vi "S_ReadProperty.vi"(8 "error in (no error)":errorcluster, 11 "reference in":refnum<class "SubTemplate_4x4x4.lvclass">) -> (0 "error out":errorcluster, 2 "property":dbl, 3 "reference out":refnum<class "SubTemplate_4x4x4.lvclass">)   [LabVIEW 2012]
uses:
  <resource>/Framework/Providers/Open_GDS/ClassProviders/Provider_EndevoGOOP300/Templates/SubTemplate_4x4x4/SubTemplate_4x4x4.lvclass
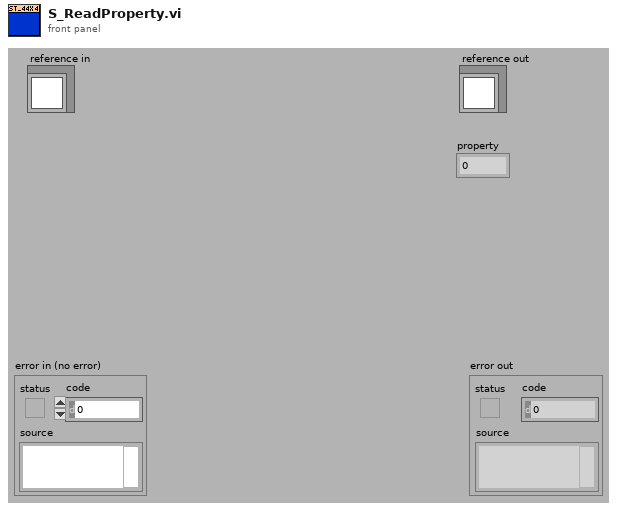
[diagram p1: front panel]
types:
  T1 = typedef "SubTemplate_4x4x4.lvclass/ObjectAttributes.ctl" = cluster{"Base class":T2}
  T2 = typedef "BaseTemplate_4x4x4.lvclass/ObjectAttributes.ctl" = cluster{"Attribute1":dbl}
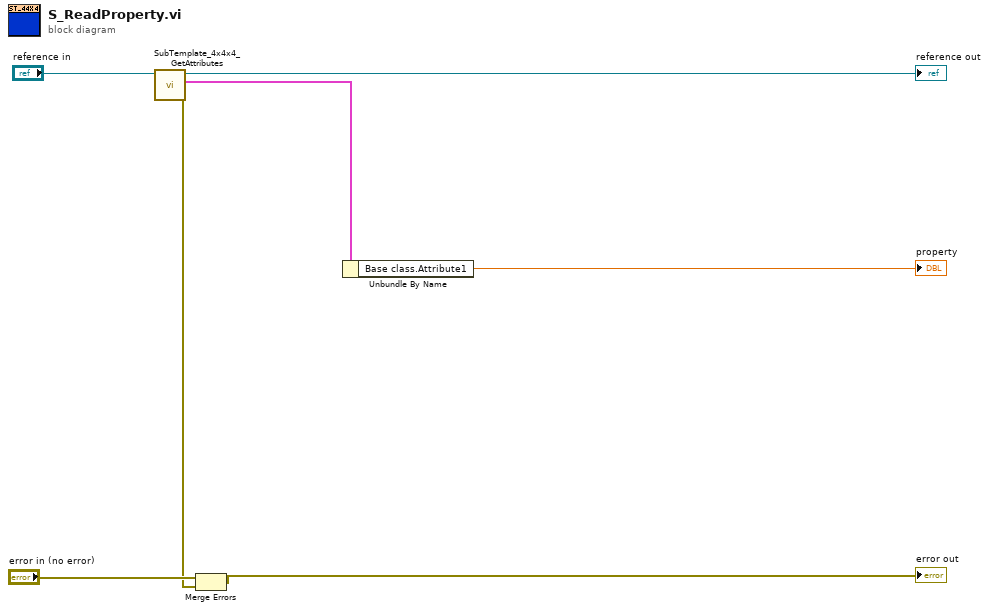
[diagram p0: block diagram]
diagram:
  n1 = call <resource>:"SubTemplate_4x4x4_GetAttributes.vi"("reference in"="reference in") -> ("error out"=w2:errorcluster, "Attributes"=w4:T1, "reference out"=→"reference out":refnum<class "SubTemplate_4x4x4.lvclass">)  [unwired: 7 in, 1 out]
  n2 = Merge Errors("error in (no error)", w2) -> (→"error out":errorcluster)
  n3 = Unbundle By Name(w4) -> ("Base class.Attribute1"=→"property":dbl)
